vi "2ndContollerStatus.vi"() -> ()   [LabVIEW 2016]
panel:
  out "status":dbl
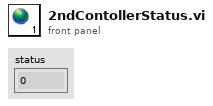
[diagram p1: front panel]
diagram:
